vi "Button Handler.vi"(8 "error in (no error)":errorcluster, 11 "Buttons":bool[](array[boolean])) -> (0 "error out":errorcluster)   [LabVIEW 2015]
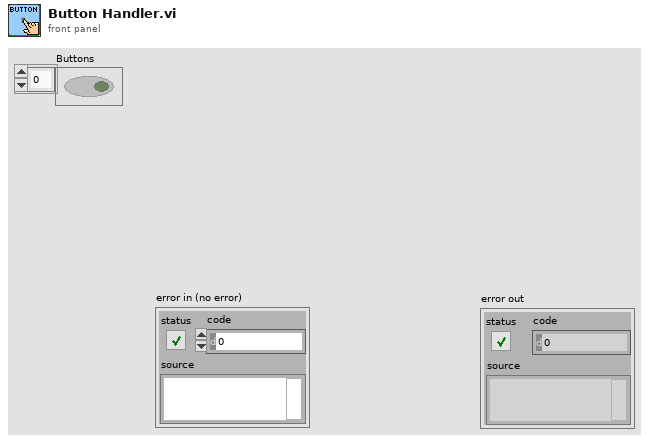
[diagram p1: front panel]
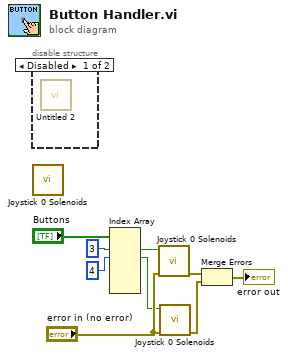
[diagram p0: block diagram]
diagram:
  n1 = disable-structure shown="Disabled" {
    frame Disabled {
      n2 = call "Untitled 2.vi"() -> ()  [unwired: 11 in, 1 out]
    }
    frame Enabled {
    }
  }
  n3 = call "Joystick 0 Solenoids.vi"() -> ()  [unwired: 11 in, 1 out]
  n4 = Index Array(array="Buttons", index #1=3 ("index"), index #2=4 ("index")) -> (element #1=w5:bool, element #2=w1:bool)  [unwired: 4 in, 4 out]
  n5 = call "Joystick 0 Solenoids.vi"("error in (no error)"="error in (no error)", "button value"=w5) -> ("error out"=w4:errorcluster)  [unwired: 9 in]
  n6 = call "Joystick 0 Solenoids.vi"("error in (no error)"="error in (no error)", "button value"=w1) -> ("error out"=w2:errorcluster)  [unwired: 9 in]
  n7 = Merge Errors(w4, w2) -> (→"error out":errorcluster)
